vi "Gen_audio_signal.vi"() -> ()   [LabVIEW 2024]
uses:
  <vilib>/sound2/lvsound2.llb/Sampling Mode.ctl
  <vilib>/sound2/lvsound2.llb/Sound Data Format.ctl
  <vilib>/sound2/lvsound2.llb/Sound Output Write (DBL Single).vi
  <vilib>/measure/NI_MABase.lvlib
panel:
  in  "Radio Buttons":enum32{"Sinusoide", "Onda quadra"}(radio)
  in  "STOP":bool
  out "Waveform Graph":waveform(dbl)(graph)
  in  "Amplitude":dbl(knob) scale=0.0..10.0
  in  "Frequency (Hz)":dbl(knob) scale=0.0..10000.0
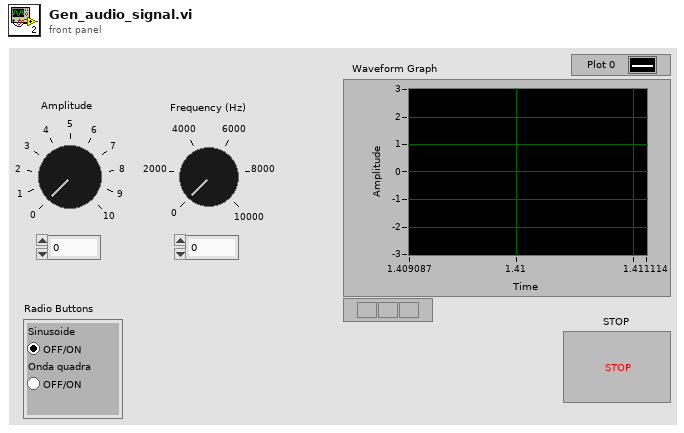
[diagram p1: front panel]
types:
  T1 = typedef "Sound Data Format.ctl" = cluster{"sample rate (S/s)":dbl, "number of channels":i32, "bits per sample":i32}
  T2 = typedef "Sampling Mode.ctl" = i32
  T3 = typedef "Sound Output Task ID.ctl" = u32
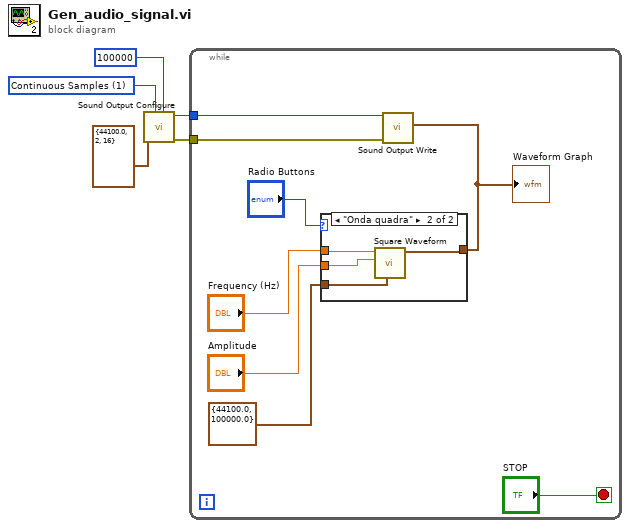
[diagram p0: block diagram]
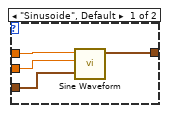
[diagram p2: hidden frame]
diagram:
  w5 = T2 1 items=["Finite Samples", "Continuous Samples"] ("sample mode")
  n1 = call <vilib>:"Sound Output Configure.vi"("number of samples/ch"=100000, "sample mode"=w5, "sound format"=T1 {"sample rate (S/s)"=44100.0, "number of channels"=2, "bits per sample"=16}) -> ("error out"=w2:errorcluster, "task ID"=w1:T3)  [unwired: 7 in]
  n2 = while {
    tunnel: w2 -> [w13]
    tunnel: w1 -> [w12]
    stop <- "STOP" stop-if-true
    n3 = case shown="\"Onda quadra\"" "Radio Buttons" {
      tunnel: "Amplitude" -> [w17 w20]
      tunnel: "Frequency (Hz)" -> [w16 w19]
      tunnel: cluster{"Fs":dbl, "#s":dbl} {"Fs"=44100.0, "#s"=100000.0} ("sampling info") -> [w15 w18]
      tunnel: [w14 w21] -> w8
      frame "Sinusoide", Default {
        n4 = call <vilib>:"Sine Waveform.vi"("sampling info"=w15, "amplitude"=w17, "frequency"=w16) -> ("signal out"=w14:waveform(dbl))  [unwired: 7 in, 1 out]
      }
      frame "Onda quadra" {
        n5 = call <vilib>:"Square Waveform.vi"("sampling info"=w18, "amplitude"=w20, "frequency"=w19) -> ("signal out"=w21:waveform(dbl))  [unwired: 7 in, 1 out]
      }
    }
    "Waveform Graph" <- w8
    n6 = call-poly <vilib>:"Sound Output Write.vi"("error in (no error)"=w13, "data"=w8, "task ID"=w12) -> ()  [unwired: 7 in, 2 out]
  }
